vi "IsWaveformDoneYet.vi"(0 "board in":u16 format="%.0x", 5 "data":u16[][](array[numeric]) format="%.0x", 11 "error in (no error)":errorcluster) -> (4 "board out":u16 format="%.0x", 6 "waveform done?":bool, 15 "error out":errorcluster)   [LabVIEW 2009, in "Hardware.lvlib" / "Channels.lvlib" / "DIO64Output.lvclass"]
doc: "This VI returns true once the output waveform has completed. It accomodates waiting around for the start trigger condition and the amount of time that the waveform itself needs. Useful to know when you need to issue a \"stop\" in software."
uses:
  DIO64Output.lvclass
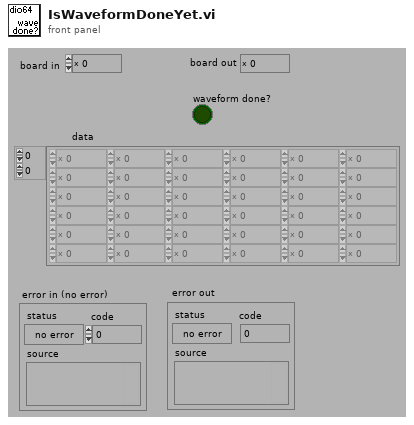
[diagram p1: front panel]
types:
  T1 = typedef "DIO64 Out Status.ctl" = cluster{"pktsize":u16, "portCount":u16, "writePtr":u16, "readPtr":u16, "time0":u16, "time1":u16, "fifoSize":u32, "fifo0":u16, "ticks":u32, "flags":u16, "clkControl":u16, "startControl":u16, "stopControl":u16, "AIControl":u32, "AICurrent":u16, "startTime0":u16, "startTime1":u16, "stopTime0":u16, "stopTime1":u16, "cur trans":u32, "cur reps":u32}
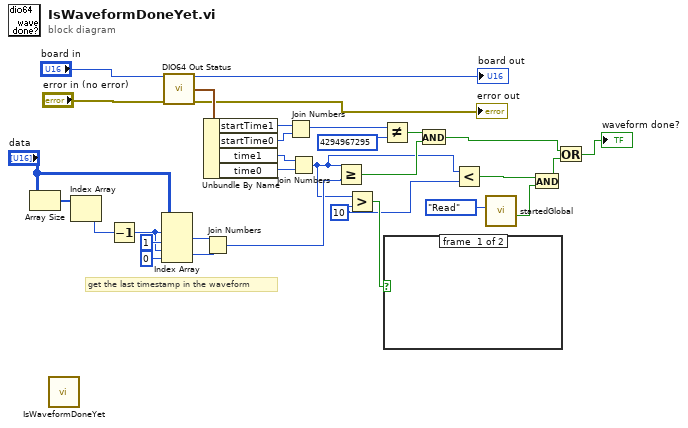
[diagram p0: block diagram]
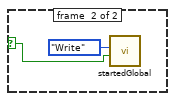
[diagram p2: hidden frame]
diagram:
  w6 = 10
  # "get the last timestamp in the waveform"
  n1 = Array Size(array="data") -> (size(s)=w21:i32[])
  n2 = call <userlib>:"IsWaveformDoneYet.vi"() -> ()  [unwired: 13 in, 3 out]
  n3 = Index Array(array=w21) -> (element=w19:i32)  [unwired: 1 in]
  n4 = Decrement(x=w19) -> (x-1=w13:i32)
  n5 = Index Array(array="data", index (row) #1=w13, index (col) #1=1 ("disabled index (col)"), index (row) #2=w13, index (col) #2=0 ("index (col)")) -> (element #1=w16:u16, element #2=w15:u16)
  n6 = call <userlib>:"DIO64 Out Status.vi"("board in"="board in", "error in (no error)"="error in (no error)") -> ("board out"=→"board out":u16, "Out Status"=w26:T1, "error out"=→"error out":errorcluster)  [unwired: 10 in, 1 out]
  n7 = Join Numbers(hi=w16, lo=w15) -> ((hi.lo)=w14:u32)
  n8 = Unbundle By Name(w26) -> ("startTime1"=w27:u16, "startTime0"=w28:u16, "time1"=w12:u16, "time0"=w11:u16)
  n9 = Join Numbers(hi=w27, lo=w28) -> ((hi.lo)=w30:u32)
  n10 = Join Numbers(hi=w12, lo=w11) -> ((hi.lo)=w7:u32)
  n11 = Greater Or Equal?(x=w7, y=w14) -> (x >= y?=w10:bool)
  n12 = Greater?(x=w7, y=w6) -> (0:w9:bool)
  n13 = Not Equal?(x=w30, y=u32 4294967295) -> (x != y?=w31:bool)
  n14 = case shown="True" w9 {
    selector: w9 -> [_ w32]
    frame #0 {
    }
    frame #1 {
      n15 = call "startedGlobal.vi"("started"=w32, "Action"=enum16{"Write", "Read", "Reset"}."Write") -> ()  [unwired: 9 in, 1 out]
    }
  }
  n16 = And(x=w31, y=w10) -> (x .and. y?=w2:bool)
  n17 = Less?(x=w7, y=w6) -> (x < y?=w5:bool)
  n18 = call "startedGlobal.vi"("Action"=enum16{"Write", "Read", "Reset"}."Read") -> ("started?"=w4:bool)  [unwired: 10 in]
  n19 = And(x=w5, y=w4) -> (x .and. y?=w3:bool)
  n20 = Or(x=w2, y=w3) -> (x .or. y?=→"waveform done?":bool)
